vi "Get Controls.vi"(0 "Diagram in":refnum<vi>, 5 "Control Names":string[](array[string]), 11 "error in (no error)":errorcluster) -> (4 "Diagram out":refnum<vi>, 6 "Control Terminals":refnum<vi>[](array[refnum]), 15 "error out":errorcluster)   [LabVIEW 2015, in "Scripting.lvlib"]
doc: "<B>Control Terminals</B> is an array of the output terminals of the controls selected with <B>Control Names</b> on <B>Diagram in</B>."
uses:
  Scripting.lvlib
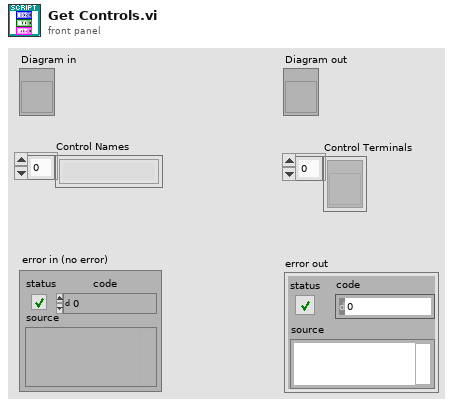
[diagram p1: front panel]
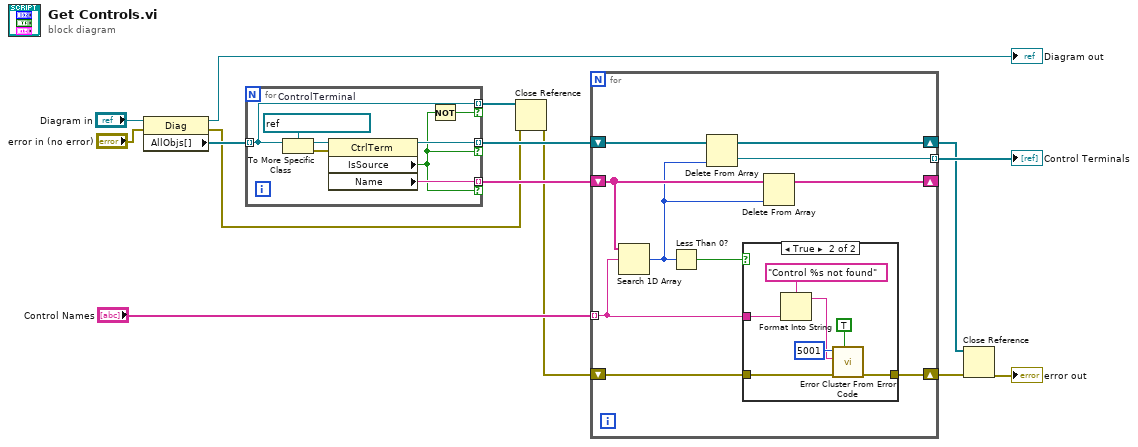
[diagram p0: block diagram]
diagram:
  n1 = property class="Diag"(reference="Diagram in", error in="error in (no error)") -> (reference out=→"Diagram out":refnum<vi>, error out=w5:errorcluster, "AllObjs[]"=w11:refnum<vi>[])
  n2 = for {
    tunnel: w11 -> [w16] mode=indexing
    tunnel: [w19] -> w10 mode=indexing if=w17
    tunnel: [w18] -> w9 mode=indexing if=w17
    tunnel: [w16] -> w6 mode=indexing if=w15
    w22 = refnum<vi> refnum  # ControlTerminal
    n3 = To More Specific Class(target class=w22, reference=w16) -> (specific class reference=w21:refnum<vi>, error out=w20:errorcluster)  [unwired: 1 in]
    n4 = property class="CtrlTerm"(reference=w21, error in=w20) -> (reference out=w19:refnum<vi>, "IsSource"=w17:bool, "Name"=w18:string)  [unwired: 1 out]
    n5 = Not(x=w17) -> (.not. x?=w15:bool)
  }
  n6 = Close Reference(reference=w6, error in (no error)=w5) -> (error out=w4:errorcluster)
  n7 = for {
    tunnel: "Control Names" -> [w29] mode=indexing
    shift-right: [w28] -> w2
    shift-left: w4 -> [w30]
    tunnel: [w27] -> w7 mode=indexing
    shift-right: [w25] -> _
    shift-left: w9 -> [w26]
    shift-right: [w23] -> w3
    shift-left: w10 -> [w32]
    n8 = Search 1D Array(1D array=w26, element=w29) -> (index of element=w24:i32)  [unwired: 1 in]
    n9 = Less Than 0?(x=w24) -> (x < 0?=w31:bool)
    n10 = Delete From Array(array=w32, index=w24) -> (deleted portion=w27:refnum<vi>, array with subset deleted=w23:refnum<vi>[])  [unwired: 1 in]
    n11 = case shown="True" w31 {
      tunnel: w30 -> [w33 w39]
      tunnel: w29 -> [_ w37]
      tunnel: [w33 w34] -> w28
      frame False {
      }
      frame True {
        n12 = Format Into String(format string="Control %s not found", w37) -> (resulting string=w36:string)  [unwired: 2 in, 1 out]
        n13 = call <vilib>:"Error Cluster From Error Code.vi"("show call chain? (False)"=TRUE, "error in (no error)"=w39, "error message (\"\")"=w36, "error code (0)"=5001) -> ("error out"=w34:errorcluster)  [unwired: 5 in]
      }
    }
    n14 = Delete From Array(array=w26, index=w24) -> (array with subset deleted=w25:string[])  [unwired: 1 in, 1 out]
  }
  "Control Terminals" <- w7
  n15 = Close Reference(reference=w3, error in (no error)=w2) -> (error out=→"error out":errorcluster)
